vi "BeamformerGUI_GivenFreqs.vi"() -> ()   [LabVIEW 2017]
uses:
  <vilib>/userdefined/High Color/IMAQdx.ctl
  <vilib>/UPVI/lvhdf5/dataset.llb/LVH5D Operation.ctl
  <vilib>/Utility/miscctls.llb/LVRectTypeDef.ctl
  <vilib>/UPVI/lvhdf5/attribute.llb/LVH5A Operation.ctl
  <vilib>/UPVI/lvhdf5/group.llb/H5G_obj_t.ctl
  <vilib>/UPVI/lvhdf5/file.llb/LVH5F Operation.ctl
  15de898c-7c44-4598-bed2-ace033be772a.vi
  <vilib>/UPVI/lvhdf5/identifier.llb/Not an HDF5 Refnum Constant.vi
  <vilib>/UPVI/lvhdf5/common.llb/To HDF5 Ref.vi
  <vilib>/measure/maspectr.llb/FFT Power Spectrum and PSD for 1 Chan.vi
  <vilib>/UPVI/lvhdf5/file.llb/OpenCreateReplace HDF5 File.vi
  <vilib>/UPVI/lvhdf5/utility.llb/Select HDF5 Dialog.vi
  <vilib>/UPVI/lvhdf5/utility.llb/Select HDF5 Dialog (File and Object).vi
  <vilib>/UPVI/lvhdf5/dataset.llb/Simple H5Dwrite (Variant).vi
  <vilib>/UPVI/lvhdf5/attribute.llb/Write Multiple Attributes.vi
  <vilib>/UPVI/lvhdf5/dataset.llb/H5Dclose.vi
  <vilib>/UPVI/lvhdf5/dataset.llb/Write Dataset with Attributes.xnode
  <vilib>/UPVI/lvhdf5/library.llb/HDF5 Ref.ctl
  <vilib>/vision/driver/NI_Vision_Acquisition_Software.lvlib
  <vilib>/Utility/error.llb/Error Cluster From Error Code.vi
  <vilib>/UPVI/lvhdf5/dataset.llb/OpenCreateReplace Dataset by Element Type.vi
  <vilib>/UPVI/lvhdf5/dataspace.llb/H5Sselect_hyperslab.vi
  <vilib>/UPVI/lvhdf5/dataset.llb/H5Dwrite (Variant).vi
  <vilib>/UPVI/lvhdf5/dataset.llb/H5Dget_space.vi
  <vilib>/UPVI/lvhdf5/attribute.llb/private/LVH5AwriteWDTAttrs.vi
  <vilib>/UPVI/lvhdf5/dataspace.llb/H5Sclose.vi
  <vilib>/Utility/VariantDataType/GetClusterInfo.vi
  <vilib>/Utility/VariantDataType/VariantType.lvlib
  <vilib>/Utility/VariantDataType/GetTypeInfo.vi
  <vilib>/UPVI/lvhdf5/attribute.llb/Cluster to Attribute Array.xnode
  <vilib>/measure/NI_MAPro.lvlib
  <vilib>/UPVI/lvhdf5/utility.llb/Select HDF5 Dialog (Object Only).vi
panel:
  in  "Experiment Name 2":string="test_calib"
  out "total_samples":dbl
  out "Data out":dbl[][](array[numeric])
  out "Array":dbl[][](array[numeric])
  in  "stop":bool
  in  "Tab Control":enum32{"Measurement", "Processing"}(tab)
  in  "Distance to array (m)":dbl=0.5
  in  "Take":bool
  in  "Data Directory":path=path "C:/Users/Lino P/Documents/000 - USFQ/TesisProd/data"
  in  "Record Data":bool
  in  "Sampling Freq. (Hz)":dbl=51200.0
  in  "Sampling Time (s)":dbl=10.0
  in  "Experiment Name":string="test_"
  in  "Audio Preview":bool
  out "Image Out":T1(plugin-control)
  in  "Session In":T2 caption="Camera"
  out "Img Ready":bool caption="Capturing Image"
  out "data":dynamicdata(graph)
  in  "Map Threshold":dbl=5.0
  out "Success":bool
  out "Server Running":bool
  out "Processing":bool
  in  "Preview Read Signal":bool
  in  "Scripts Directory":path=path "C:/Users/Lino P/Documents/000 - USFQ/TesisDev/py"
  in  "Lower":dbl=3000.0
  in  "Microphone Geometry":path=path "C:/Users/Lino P/Documents/000 - USFQ/TesisProd/data/xml/16_mics_geom.xml"
  out "Info":string
  out "Warnings":string
  out "Return Code":dbl
  out "Error":bool
  in  "Audio Data File (HDF5)":path=path "C:/Users/Lino P/Documents/000 - USFQ/TesisProd/data/test_exe.h5"
  in  "RunAnalysis":bool
  out "Selected Mic":dbl[](graph)
  out "Frequency Domain":cluster{"f0":dbl, "df":dbl, "magnitude":dbl[]}(graph)
  out "Sampling Freq. (Hz)":dbl
  in  "Higher":dbl=5000.0 caption="high_freq"
  in  "Channel":u16(ring) items=["1", "2", "3", "4", "5", "6", "7", "8", "9", "10", "11", "12", "13", "14", "15", "16"]
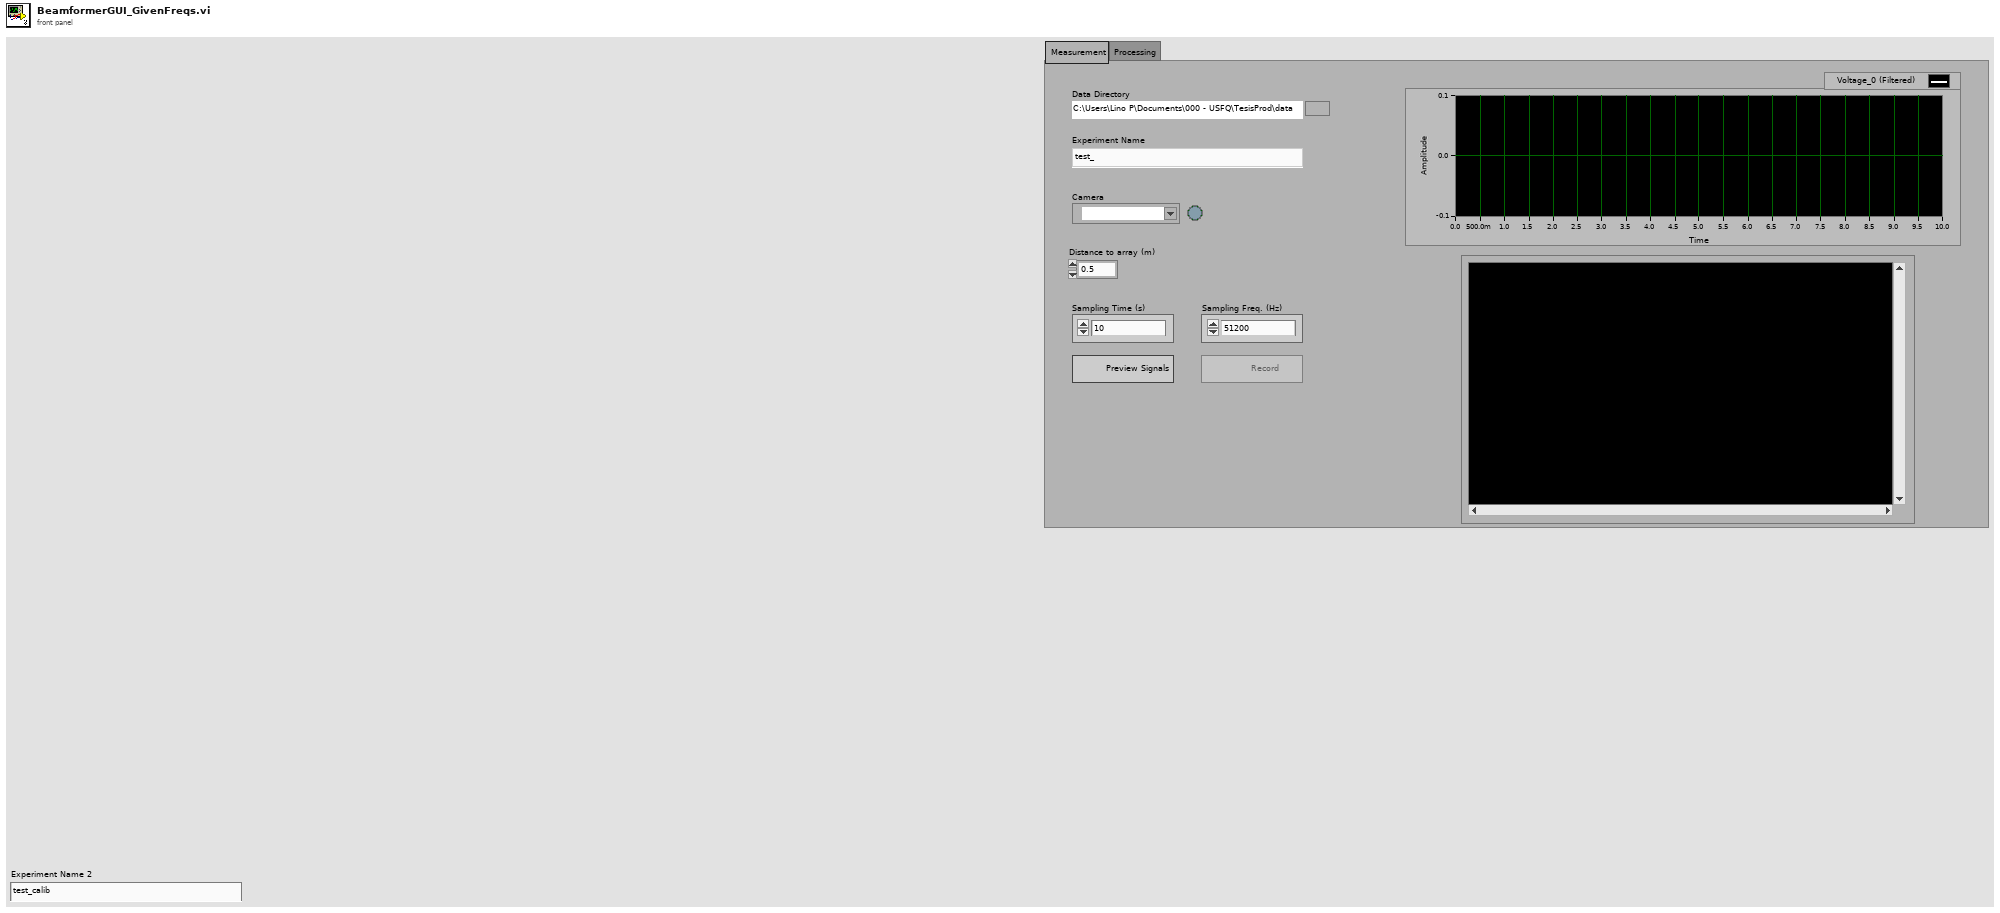
[diagram p1: front panel]
types:
  T1 = typedef "IMAQ Image.ctl" = refnum<image>
  T2 = typedef "IMAQdx.ctl" = refnum<k21>
  T3 = enum8{"Enabled", "Disabled", "Disabled and Grayed Out"}
  T4 = typedef "Image Type" = u32
  T5 = typedef "LVH5D Operation.ctl" = enum16{"open", "replace", "create", "open or create", "create or replace", "create or replace with confirmation"}
  T6 = typedef "LVH5A Operation.ctl" = enum16{"open", "replace", "create", "open or create", "create or replace", "create or replace with confirmation"}
  T7 = typedef "LVRectTypeDef.ctl" = cluster{"Left":i16, "Top":i16, "Right":i16, "Bottom":i16}
  T8 = cluster{"Behavior":enum32{"Invalid", "Default", "Floating", "Floating/Auto-Hide", "Modal"}, "Position":T7, "Center":bool, "Title":string}
  T9 = typedef "LVH5F Operation.ctl" = enum16{"open", "open or create", "create or replace", "create or replace (with confirmation)", "create", "open (read only)"}
  T10 = typedef "H5G_obj_t.ctl" = i32
  T11 = cluster{"Object Types (any)":T10[], "Object Pattern":string}
  T12 = enum32{"Invalid", "Standard", "Closed", "Hidden", "Minimized", "Maximized"}
  T13 = typedef "HDF5 Ref.ctl" = refnum<k1>
  T14 = cluster{"Left":i32, "Top":i32, "Right":i32, "Bottom":i32}
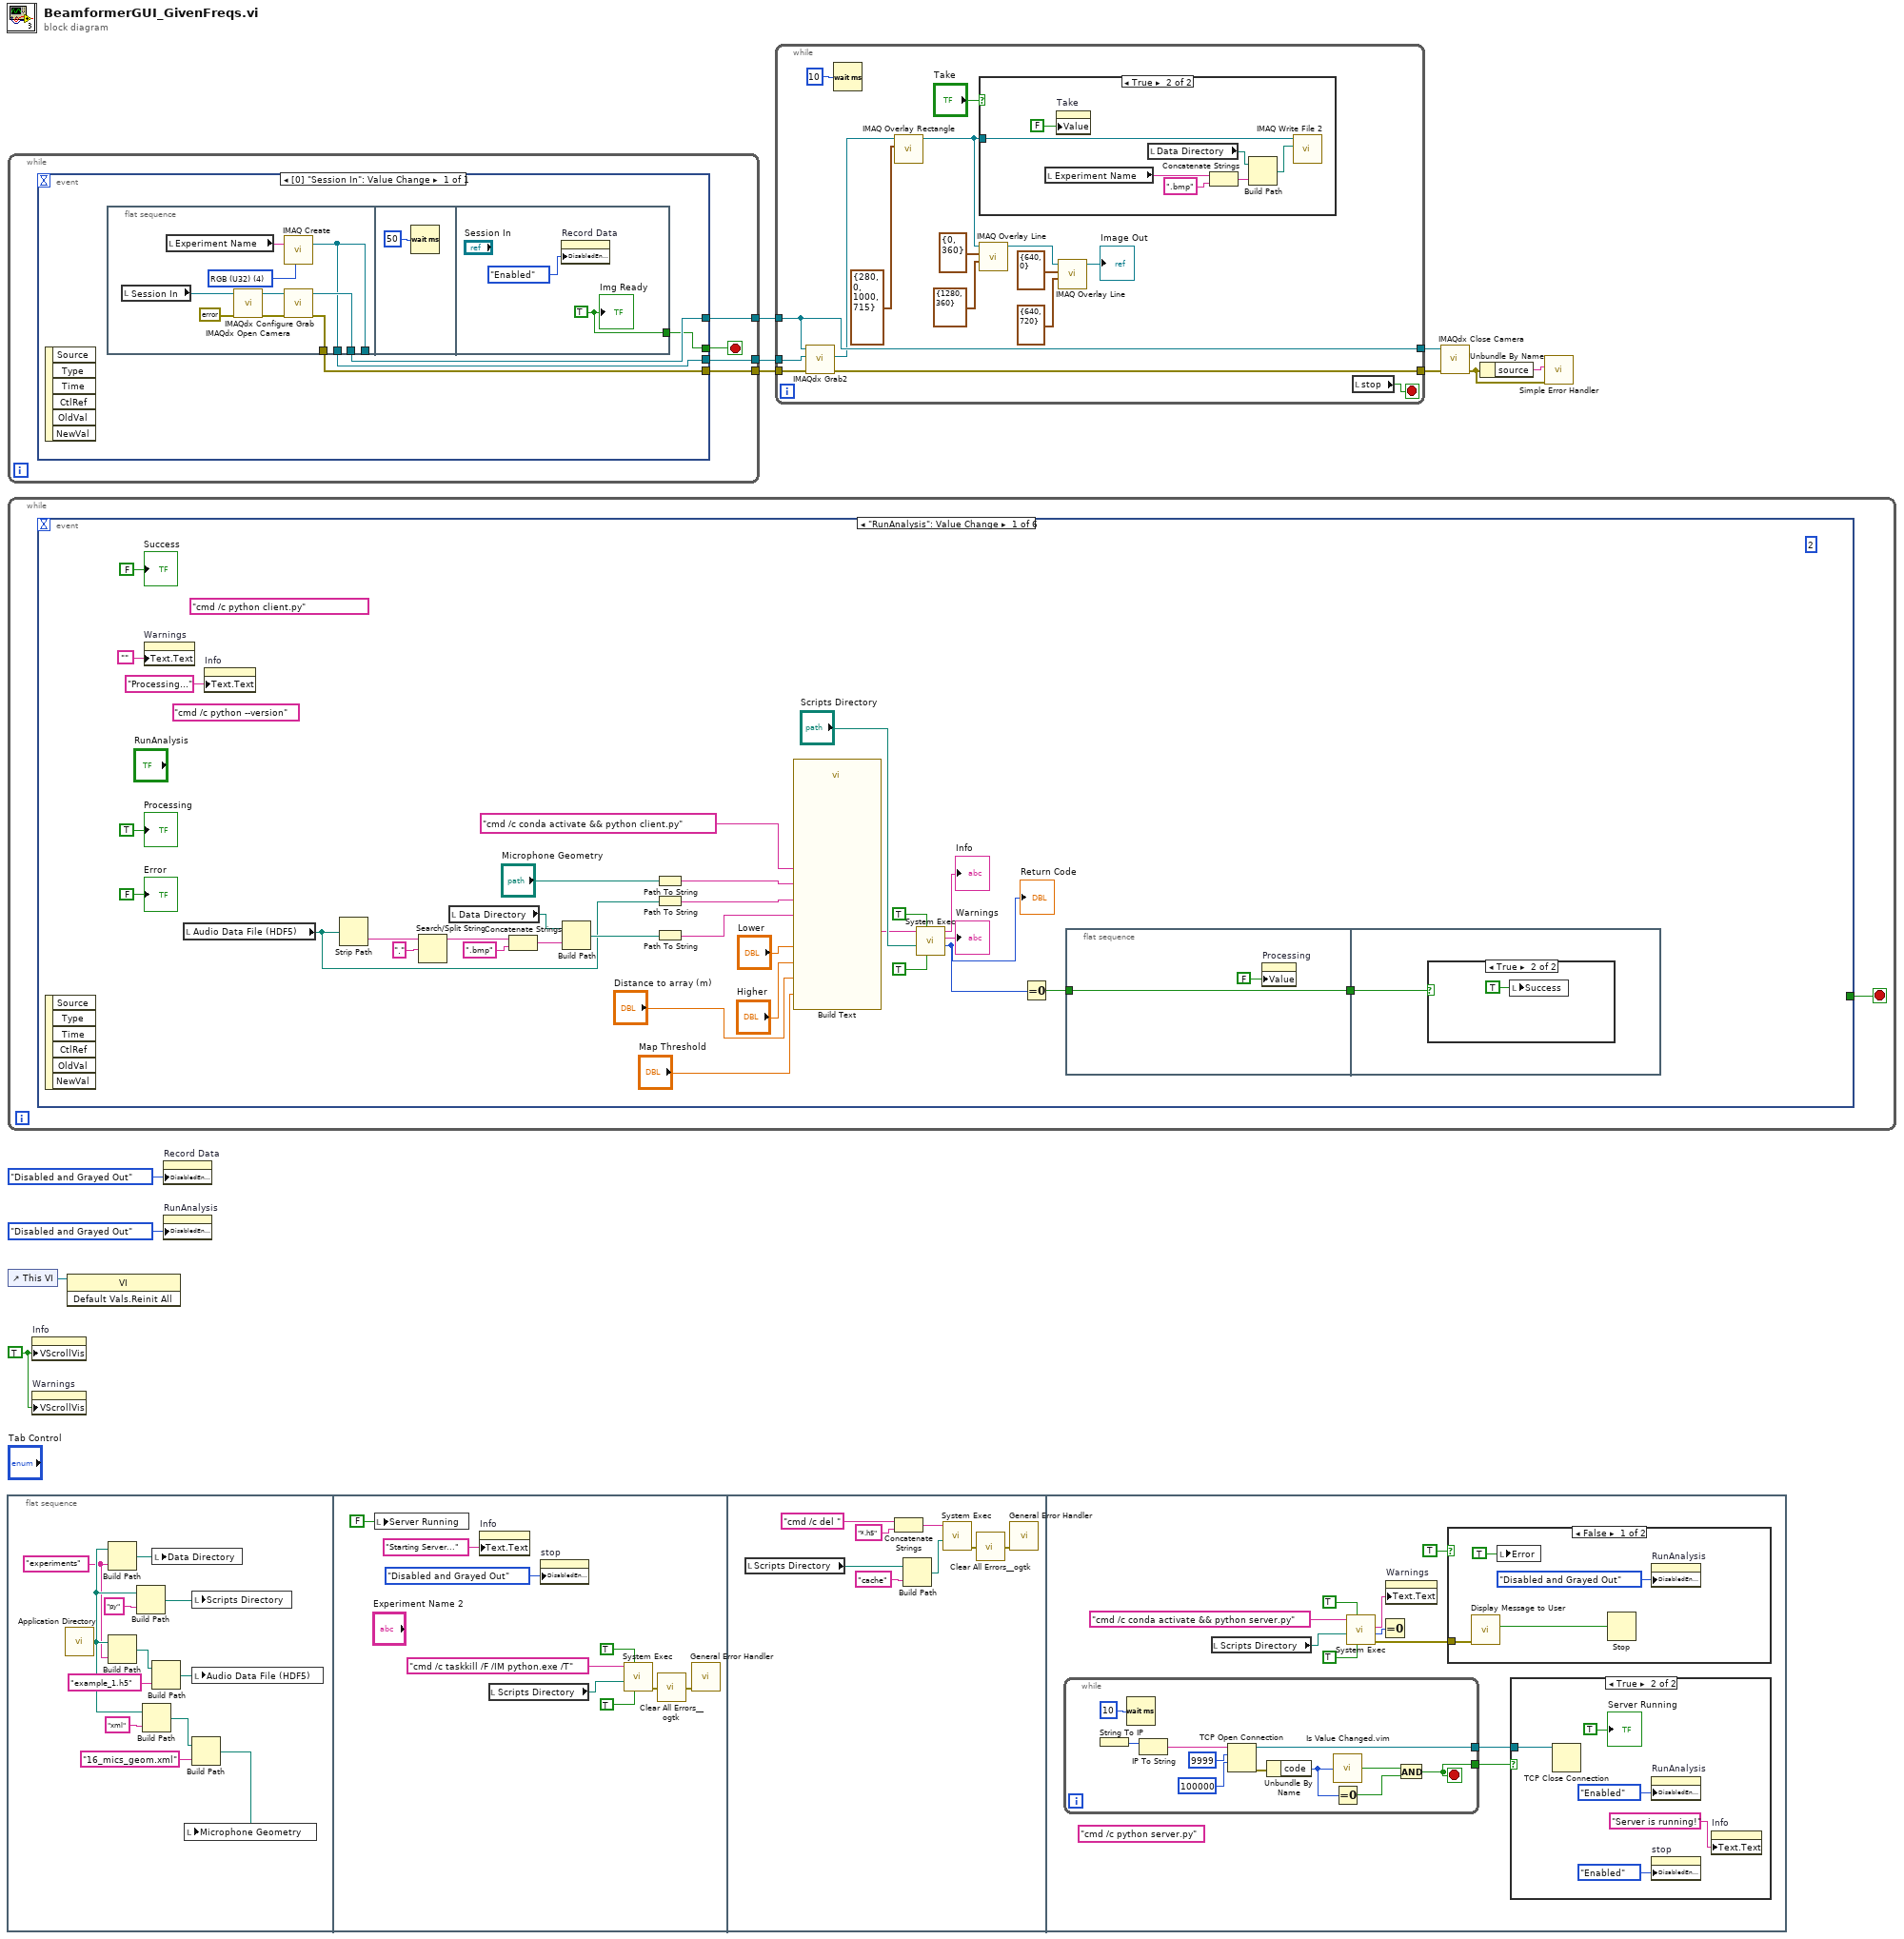
[diagram p0: block diagram]
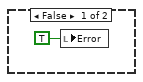
[diagram p5: hidden frame]
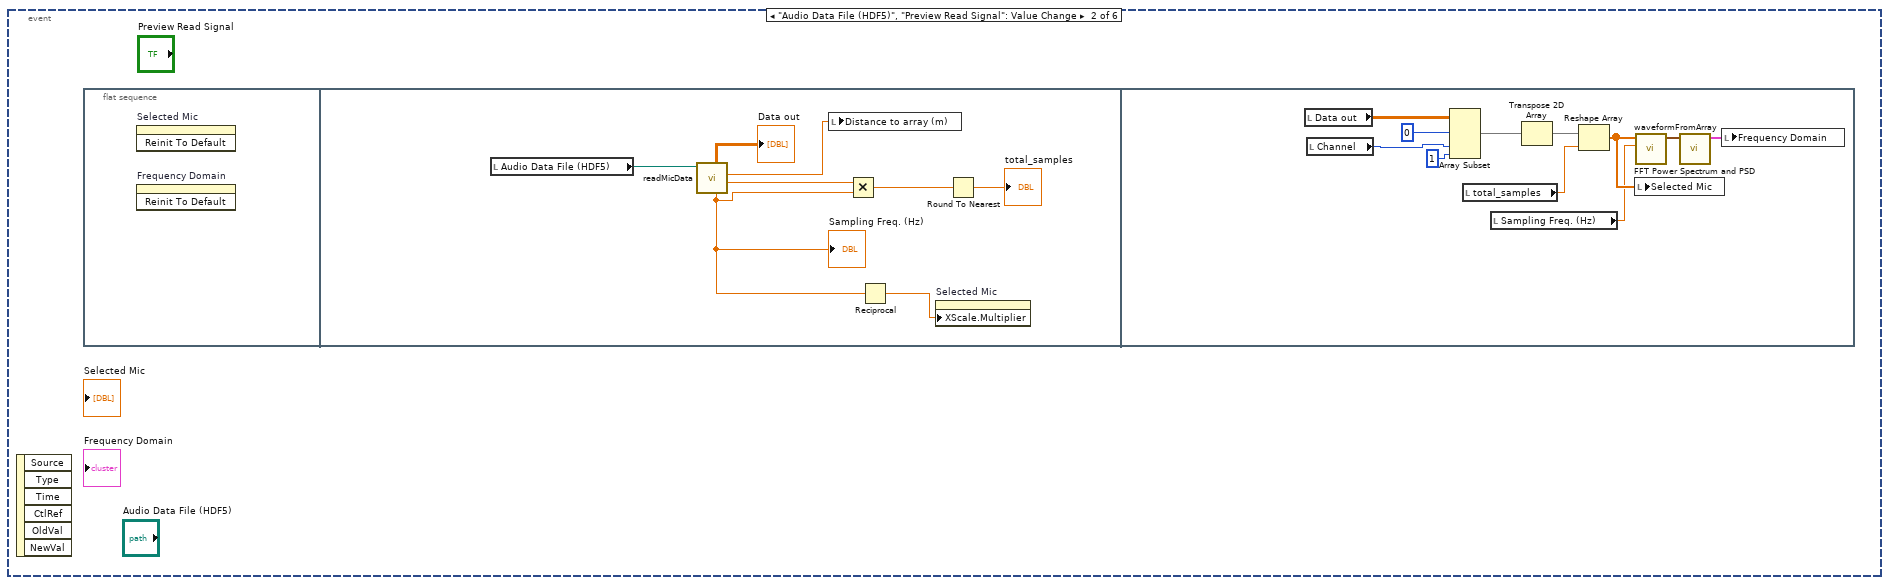
[diagram p6: hidden frame]
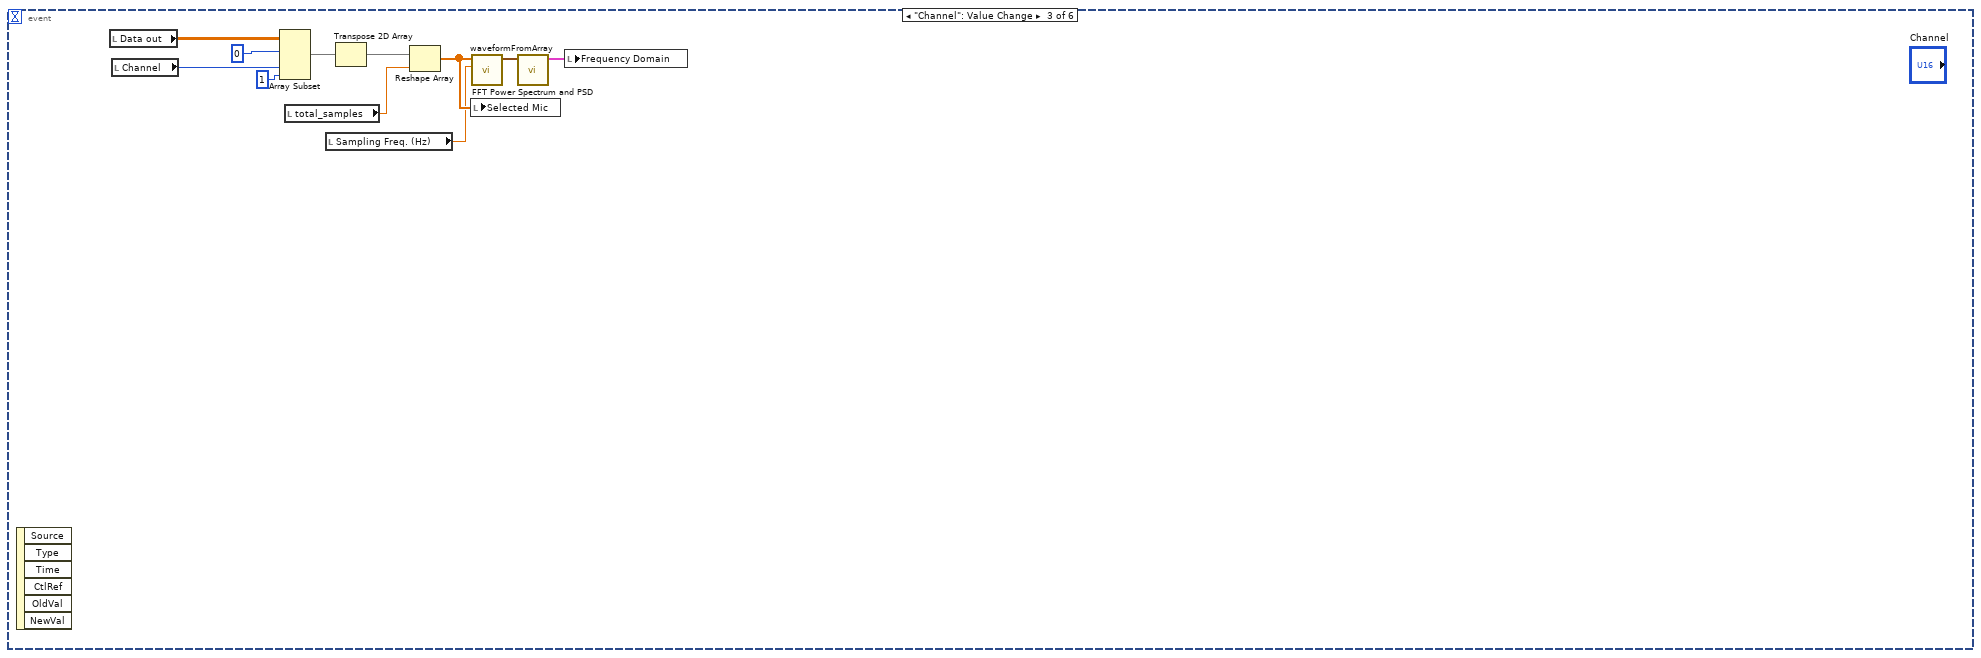
[diagram p7: hidden frame]
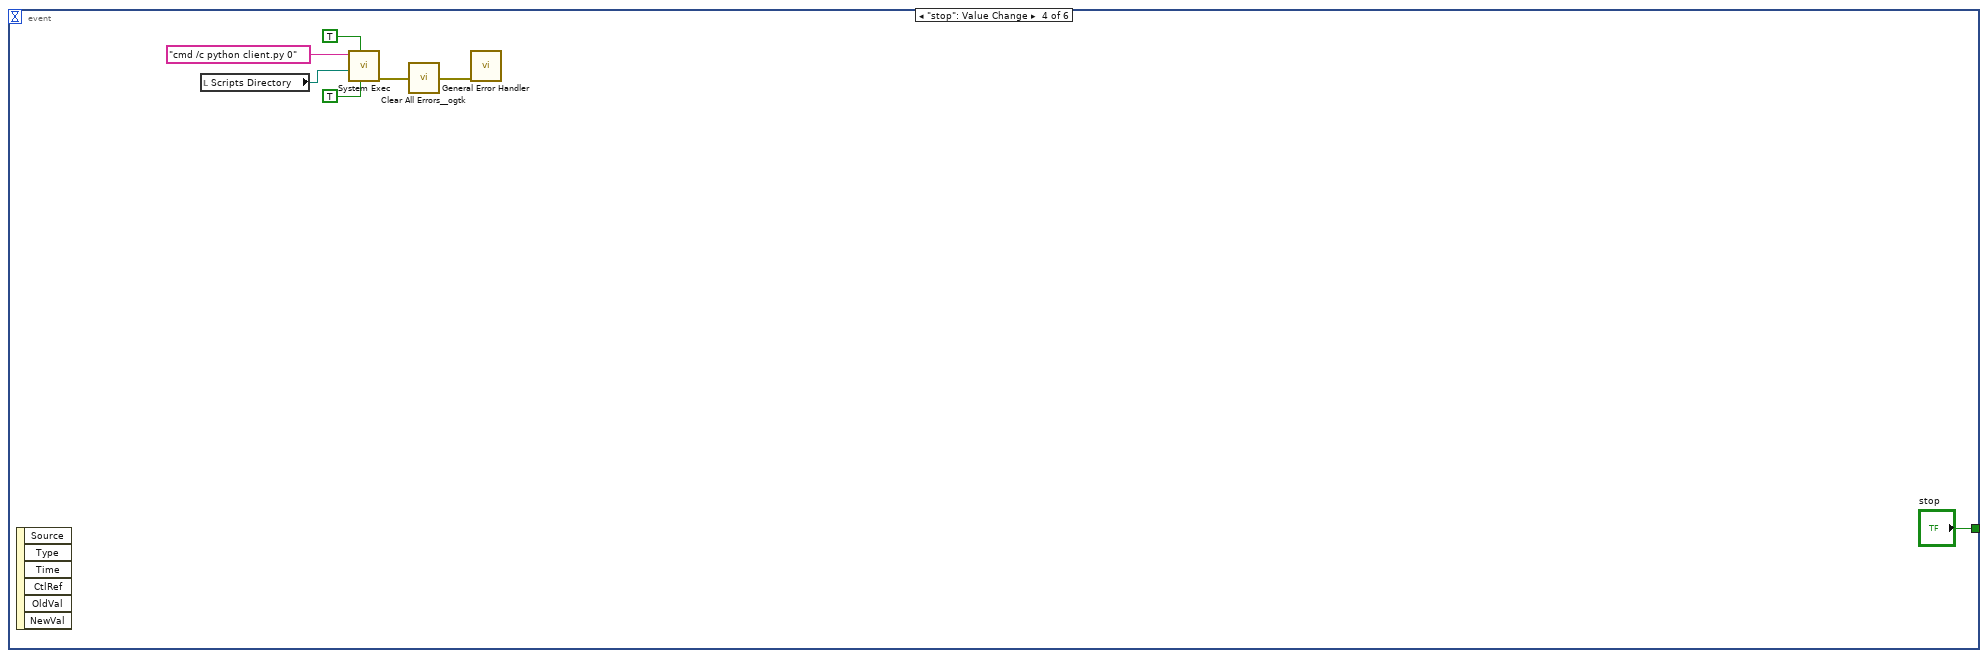
[diagram p8: hidden frame]
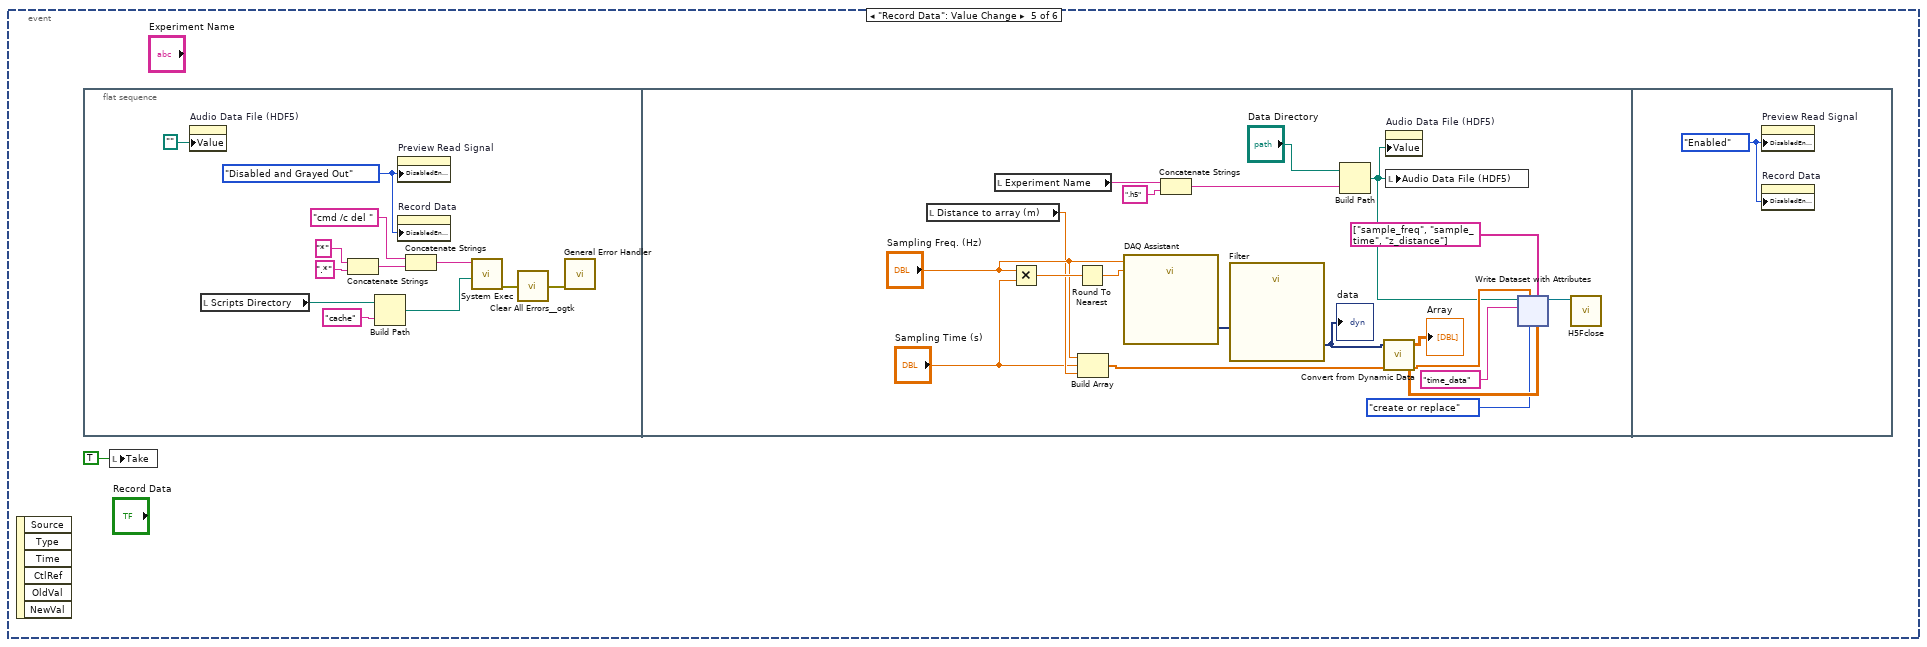
[diagram p9: hidden frame]
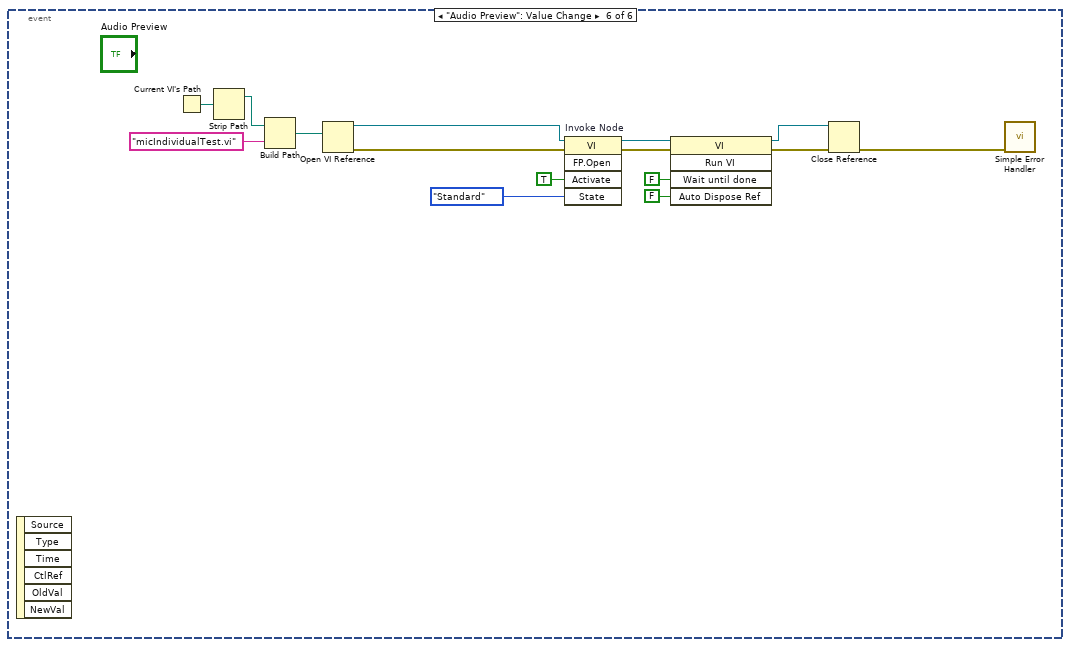
[diagram p10: hidden frame]
diagram:
  w10 = TRUE
  n1 = flat-sequence {
    frame #0 {
      w16 = "experiments" ("name or relative path")
      n2 = call <vilib>:"Application Directory.vi"() -> ("Application Directory"=w19:path)
      n3 = Build Path(base path=w19, name or relative path=w16) -> (appended path=w20:path)
      n4 = Build Path(base path=w19, name or relative path=w16) -> (appended path=w15:path)
      n5 = Build Path(base path=w19, name or relative path="py") -> (appended path=w22:path)
      n6 = Build Path(base path=w19, name or relative path="xml") -> (appended path=w18:path)
      n7 = local write "Data Directory"(w20) -> ()
      n8 = Build Path(base path=w15, name or relative path="example_1.h5") -> (appended path=w13:path)
      n9 = local write "Scripts Directory"(w22) -> ()
      n10 = local write "Audio Data File (HDF5)"(w13) -> ()
      n11 = Build Path(base path=w18, name or relative path="16_mics_geom.xml") -> (appended path=w12:path)
      n12 = local write "Microphone Geometry"(w12) -> ()
    }
    frame #1 {
      n13 = local write "Server Running"(FALSE ("Server Running")) -> ()
      n14 = property on="Info" class="Str"("Text.Text"="Starting Server...") -> ()  [unwired: 2 in, 2 out]
      n15 = local read "Scripts Directory"() -> (w32:path)
      n16 = property on="stop" class="Bool (strict)"("DisabledEnum"=T3."Disabled and Grayed Out" ("Disabled")) -> ()  [unwired: 2 in, 2 out]
      n17 = call <vilib>:"System Exec.vi"("run minimized? (F)"=TRUE, "wait until completion? (T)"=TRUE, "working directory"=w32, "command line"="cmd /c taskkill /F /IM python.exe /T") -> ("error out"=w28:errorcluster)  [unwired: 4 in, 3 out]
      n18 = call <userlib>:"Clear All Errors__ogtk.vi"("Error In"=w28) -> ("Error Out"=w29:errorcluster)  [unwired: 3 in]
      n19 = call <vilib>:"General Error Handler.vi"("error in (no error)"=w29) -> ()  [unwired: 10 in, 5 out]
    }
    frame #2 {
      n20 = local read "Scripts Directory"() -> (w39:path)
      n21 = Concatenate Strings("cmd /c del " ("command line"), "*.h5" ("string")) -> (w36:string)
      n22 = Build Path(base path=w39, name or relative path="cache") -> (appended path=w40:path)
      n23 = call <vilib>:"System Exec.vi"("working directory"=w40, "command line"=w36) -> ("error out"=w38:errorcluster)  [unwired: 6 in, 3 out]
      n24 = call <userlib>:"Clear All Errors__ogtk.vi"("Error In"=w38) -> ("Error Out"=w37:errorcluster)  [unwired: 3 in]
      n25 = call <vilib>:"General Error Handler.vi"("error in (no error)"=w37) -> ()  [unwired: 10 in, 5 out]
    }
    frame #3 {
      (unwired) "cmd /c python server.py" ("command line")
      n26 = while {
        tunnel: [w60] -> w42
        tunnel: [w58] -> w41
        stop <- w60 stop-if-true
        n27 = String To IP() -> (0:w56:u32)  [unwired: 1 in]
        n28 = Wait (ms)(milliseconds to wait=u32 10) -> ()  [unwired: 1 out]
        n29 = IP To String(2:w56) -> (0:w57:string)  [unwired: 1 in]
        n30 = TCP Open Connection(address=w57, remote port or service name=u16 9999, timeout ms (60000)=100000) -> (connection ID=w58:refnum<k5>, error out=w59:errorcluster)  [unwired: 2 in]
        n31 = Unbundle By Name(w59) -> ("code"=w63:i32)
        n32 = call "Is Value Changed.vim"("value"=w63) -> ("changed or first call?"=w61:bool)
        n33 = Equal To 0?(x=w63) -> (x = 0?=w62:bool)
        n34 = And(x=w61, y=w62) -> (x .and. y?=w60:bool)
      }
      n35 = local read "Scripts Directory"() -> (w47:path)
      n36 = call <vilib>:"System Exec.vi"("run minimized? (F)"=TRUE, "wait until completion? (T)"=TRUE, "working directory"=w47, "command line"="cmd /c conda activate && python server.py") -> ("error out"=w49:errorcluster, "return code"=w48:i32, "standard error"=w50:string)  [unwired: 4 in, 1 out]
      n37 = Equal To 0?(x=w48) -> ()  [unwired: 1 out]
      n38 = property on="Warnings" class="Str"("Text.Text"=w50) -> ()  [unwired: 2 in, 2 out]
      n39 = case shown="False" TRUE {
        tunnel: w49 -> [w67 _]
        frame False {
          n40 = call "Display Message to User"("error in (no error)"=w67) -> ("OK"=w68:bool)  [unwired: 9 in, 1 out]
          n41 = local write "Error"(TRUE ("Error")) -> ()
          n42 = Stop(stop? (T)=w68) -> ()
          n43 = property on="RunAnalysis" class="Bool"("DisabledEnum"=T3."Disabled and Grayed Out" ("Disabled")) -> ()  [unwired: 2 in, 2 out]
        }
        frame True {
        }
      }
      n44 = case shown="True" w42 {
        tunnel: w41 -> [_ w54]
        frame False {
        }
        frame True {
          n45 = TCP Close Connection(connection ID=w54) -> ()  [unwired: 2 in, 2 out]
          n46 = property on="RunAnalysis" class="Bool"("DisabledEnum"=T3."Enabled" ("Disabled")) -> ()  [unwired: 2 in, 2 out]
          n47 = property on="stop" class="Bool (strict)"("DisabledEnum"=T3."Enabled" ("Disabled")) -> ()  [unwired: 2 in, 2 out]
          n48 = property on="Info" class="Str"("Text.Text"="Server is running!") -> ()  [unwired: 2 in, 2 out]
          "Server Running" <- TRUE ("Server Running")
        }
      }
    }
  }
  n49 = while {
    tunnel: [w73] -> w5
    tunnel: [w74] -> w4
    tunnel: [w72] -> w1
    stop <- w71 stop-if-true
    n50 = event shown="[0] \"Session In\": Value Change" {
      selector: _ -> [_]
      dyn-events: _ -> [_]
      timeout: _ -> [_]
      tunnel: [w78] -> w74
      tunnel: [w77] -> w73
      tunnel: [w76] -> w72
      tunnel: [w75] -> w71
      event Value Change {
        n51 = event-data() -> ()  [unwired: 1 in, 6 out]
        n52 = flat-sequence {
          tunnel: [w82] -> w78
          tunnel: [w81] -> w77
          tunnel: [w79] -> w76
          tunnel: [w79] -> _
          tunnel: [w90] -> w75
          frame #0 {
            w83 = T4 4 items=["Grayscale (U8)", "Grayscale (I16)", "Grayscale (SGL)", "Complex (CSG)", "RGB (U32)", "HSL (U32)", "RGB (U64)", "Grayscale (U16)"] ("Image Type")
            n53 = local read "Session In"() -> (w87:T2)
            n54 = local read "Experiment Name"() -> (w80:string)
            n55 = call <vilib>:"IMAQdx Open Camera.vi"("error in"=errorcluster {"status"=FALSE, "code"=0, "source"=""}, "Session In"=w87) -> ("error out"=w85:errorcluster, "Session Out"=w86:T2)  [unwired: 8 in]
            n56 = call "IMAQ Create"("Image Name"=w80, "Image Type"=w83) -> ("New Image"=w79:T1)  [unwired: 3 in, 1 out]
            n57 = call <vilib>:"IMAQdx Configure Grab.vi"("error in"=w85, "Session In"=w86) -> ("error out"=w82:errorcluster, "Session Out"=w81:T2)  [unwired: 8 in]
          }
          frame #1 {
            n58 = Wait (ms)(milliseconds to wait=u32 50) -> ()  [unwired: 1 out]
          }
          frame #2 {
            w90 = TRUE
            n59 = property on="Record Data" class="Bool"("DisabledEnum"=T3."Enabled" ("Disabled")) -> ()  [unwired: 2 in, 2 out]
            "Img Ready" <- w90
          }
        }
      }
    }
  }
  n60 = while {
    stop <- w91 stop-if-true
    n61 = event shown="[0] \"RunAnalysis\": Value Change" {
      selector: _ -> [_ _ _ _ _ _]
      dyn-events: _ -> [_ _ _ _ _ _]
      timeout: _ -> [_ _ _ _ _ _]
      tunnel: [_ _ _ "stop" _ _] -> w91
      event "RunAnalysis": Value Change {
        (unwired) "cmd /c python client.py"
        (unwired) 2
        (unwired) "cmd /c python --version" ("command line")
        n62 = event-data() -> ()  [unwired: 1 in, 6 out]
        n63 = property on="Warnings" class="Str"("Text.Text"="") -> ()  [unwired: 2 in, 2 out]
        n64 = local read "Audio Data File (HDF5)"() -> (w95:path)
        n65 = property on="Info" class="Str"("Text.Text"="Processing...") -> ()  [unwired: 2 in, 2 out]
        n66 = Strip Path(path=w95) -> (name=w93:string)  [unwired: 1 out]
        n67 = Search/Split String(string=w93, search string/char (-)=".") -> (substring before match=w92:string)  [unwired: 1 in, 2 out]
        n68 = local read "Data Directory"() -> (w101:path)
        n69 = Concatenate Strings(w92, ".bmp" ("string")) -> (w100:string)
        n70 = Build Path(base path=w101, name or relative path=w100) -> (appended path=w98:path)
        n71 = Path To String(path="Microphone Geometry") -> (string=w117:string)
        n72 = Path To String(path=w95) -> (string=w116:string)
        n73 = Path To String(path=w98) -> (string=w110:string)
        n74 = call "Build Text"("image"=w110, "high_freq"="Higher", "thresh"="Map Threshold", "cmd"="cmd /c conda activate && python client.py", "mic_geo"=w117, "data"=w116, "low_freq"="Lower", "z_distance"="Distance to array (m)") -> ("Result"=w112:string)  [unwired: 6 in, 1 out]
        n75 = call <vilib>:"System Exec.vi"("run minimized? (F)"=TRUE, "wait until completion? (T)"=TRUE, "working directory"="Scripts Directory", "command line"=w112) -> ("return code"=w114:i32, "standard error"=→"Warnings":string, "standard output"=→"Info":string)  [unwired: 4 in, 1 out]
        "Return Code" <- w114
        n76 = Equal To 0?(x=w114) -> (x = 0?=w108:bool)
        n77 = flat-sequence {
          tunnel: w108 -> [w124]
          tunnel: [w124] -> w107
          tunnel: w107 -> [w125]
          frame #0 {
            n78 = property on="Processing" class="Bool (strict)"("Value"=FALSE ("Processing")) -> ()  [unwired: 2 in, 2 out]
          }
          frame #1 {
            n79 = case shown="True" w125 {
              frame False {
                n80 = local write "Error"(TRUE ("Error")) -> ()
              }
              frame True {
                n81 = local write "Success"(TRUE ("Success")) -> ()
              }
            }
          }
        }
        "Processing" <- TRUE
        "Error" <- FALSE ("Error")
        "Success" <- FALSE ("Success\nSuccess")
      }
      event "Audio Data File (HDF5)", "Preview Read Signal": Value Change {
        n82 = event-data() -> ()  [unwired: 1 in, 6 out]
        n83 = flat-sequence {
          frame #0 {
            n84 = invoke on="Selected Mic" class="WFGraph (strict)" method="Reinit To Default"() -> ()  [unwired: 3 in, 3 out]
            n85 = invoke on="Frequency Domain" class="WFGraph (strict)" method="Reinit To Default"() -> ()  [unwired: 3 in, 3 out]
          }
          frame #1 {
            n86 = local read "Audio Data File (HDF5)"() -> (w128:path)
            n87 = call "readMicData.vi"("HDF5 Path or Ref"=w128) -> ("sample_time"=w132:dbl, "z_distance"=w130:dbl, "sample_freq"=w133:dbl, "Data out"=→"Data out":dbl[][])  [unwired: 5 in, 2 out]
            "Sampling Freq. (Hz)" <- w133
            n88 = local write "Distance to array (m)"(w130) -> ()
            n89 = Multiply(x=w132, y=w133) -> (x*y=w131:dbl)
            n90 = Reciprocal(x=w133) -> (1/x=w129:dbl)
            n91 = property on="Selected Mic" class="WFGraph (strict)"("XScale.Multiplier"=w129) -> ()  [unwired: 2 in, 2 out]
            n92 = Round To Nearest(number=w131) -> (nearest integer value=→"total_samples":dbl)
          }
          frame #2 {
            n93 = local read "Data out"() -> (w143:dbl[][])
            n94 = local read "Channel"() -> (w142:u16)
            n95 = Array Subset(array=w143, index (row)=0 ("index"), index (col)=w142, length (col)=1 ("length")) -> (w144:dbl[][])  [unwired: 1 in]
            n96 = local read "total_samples"() -> (w138:dbl)
            n97 = local read "Sampling Freq. (Hz)"() -> (w139:dbl)
            n98 = Transpose 2D Array(2D array=w144) -> (transposed array=w145:dbl[][])
            n99 = Reshape Array(w145, w138) -> (w140:dbl[])
            n100 = local write "Selected Mic"(w140) -> ()
            n101 = call "waveformFromArray.vi"("sample_freq"=w139, "Array"=w140) -> ("waveform"=w146:waveform(dbl))  [unwired: 9 in]
            n102 = call-poly <vilib>:"FFT Power Spectrum and PSD.vi"("time signal"=w146) -> ("Power Spectrum / PSD"=w141:cluster{"f0":dbl, "df":dbl, "magnitude":dbl[]})  [unwired: 7 in, 3 out]
            n103 = local write "Frequency Domain"(w141) -> ()
          }
        }
      }
      event "Channel": Value Change {
        n104 = event-data() -> ()  [unwired: 1 in, 6 out]
        n105 = local read "Data out"() -> (w154:dbl[][])
        n106 = local read "Channel"() -> (w153:u16)
        n107 = Array Subset(array=w154, index (row)=0 ("index"), index (col)=w153, length (col)=1 ("length")) -> (w155:dbl[][])  [unwired: 1 in]
        n108 = local read "total_samples"() -> (w147:dbl)
        n109 = local read "Sampling Freq. (Hz)"() -> (w148:dbl)
        n110 = Transpose 2D Array(2D array=w155) -> (transposed array=w156:dbl[][])
        n111 = Reshape Array(w156, w147) -> (w149:dbl[])
        n112 = local write "Selected Mic"(w149) -> ()
        n113 = call "waveformFromArray.vi"("sample_freq"=w148, "Array"=w149) -> ("waveform"=w157:waveform(dbl))  [unwired: 9 in]
        n114 = call-poly <vilib>:"FFT Power Spectrum and PSD.vi"("time signal"=w157) -> ("Power Spectrum / PSD"=w152:cluster{"f0":dbl, "df":dbl, "magnitude":dbl[]})  [unwired: 7 in, 3 out]
        n115 = local write "Frequency Domain"(w152) -> ()
      }
      event "stop": Value Change {
        n116 = event-data() -> ()  [unwired: 1 in, 6 out]
        n117 = local read "Scripts Directory"() -> (w163:path)
        n118 = call <vilib>:"System Exec.vi"("run minimized? (F)"=TRUE, "wait until completion? (T)"=TRUE, "working directory"=w163, "command line"="cmd /c python client.py 0") -> ("error out"=w158:errorcluster)  [unwired: 4 in, 3 out]
        n119 = call <userlib>:"Clear All Errors__ogtk.vi"("Error In"=w158) -> ("Error Out"=w159:errorcluster)  [unwired: 3 in]
        n120 = call <vilib>:"General Error Handler.vi"("error in (no error)"=w159) -> ()  [unwired: 10 in, 5 out]
      }
      event "Record Data": Value Change {
        n121 = event-data() -> ()  [unwired: 1 in, 6 out]
        n122 = flat-sequence {
          frame #0 {
            w176 = T3."Disabled and Grayed Out" ("Disabled")
            n123 = property on="Audio Data File (HDF5)" class="Path"("Value"=path "") -> ()  [unwired: 2 in, 2 out]
            n124 = local read "Scripts Directory"() -> (w168:path)
            n125 = Concatenate Strings("*" ("string"), ".*" ("string")) -> (w170:string)
            n126 = Build Path(base path=w168, name or relative path="cache") -> (appended path=w167:path)
            n127 = property on="Preview Read Signal" class="Bool"("DisabledEnum"=w176) -> ()  [unwired: 2 in, 2 out]
            n128 = property on="Record Data" class="Bool"("DisabledEnum"=w176) -> ()  [unwired: 2 in, 2 out]
            n129 = Concatenate Strings("cmd /c del " ("command line"), w170) -> (w173:string)
            n130 = call <vilib>:"System Exec.vi"("working directory"=w167, "command line"=w173) -> ("error out"=w171:errorcluster)  [unwired: 6 in, 3 out]
            n131 = call <userlib>:"Clear All Errors__ogtk.vi"("Error In"=w171) -> ("Error Out"=w172:errorcluster)  [unwired: 3 in]
            n132 = call <vilib>:"General Error Handler.vi"("error in (no error)"=w172) -> ()  [unwired: 10 in, 5 out]
          }
          frame #1 {
            n133 = local read "Distance to array (m)"() -> (w192:dbl)
            n134 = local read "Experiment Name"() -> (w182:string)
            n135 = Multiply(x="Sampling Freq. (Hz)", y="Sampling Time (s)") -> (x*y=w194:dbl)
            n136 = Round To Nearest(number=w194) -> (nearest integer value=w195:dbl)
            n137 = Build Array("Sampling Freq. (Hz)", "Sampling Time (s)", w192) -> (w189:dbl[])
            n138 = call "DAQ Assistant"("rate"="Sampling Freq. (Hz)", "number of samples"=w195) -> ("data"=w179:dynamicdata)  [unwired: 15 in, 2 out]
            n139 = Concatenate Strings(w182, ".h5" ("string")) -> (w181:string)
            n140 = call "Filter"("Signal"=w179) -> ("Filtered Signal"=w178:dynamicdata)  [unwired: 9 in, 1 out]
            "data" <- w178
            n141 = Build Path(base path="Data Directory", name or relative path=w181) -> (appended path=w180:path)
            n142 = call "Convert from Dynamic Data"("Dynamic Data Type"=w178) -> ("Array"=w190:dbl[][])  [unwired: 3 in]
            "Array" <- w190
            n143 = property on="Audio Data File (HDF5)" class="Path"("Value"=w180) -> ()  [unwired: 2 in, 2 out]
            n144 = local write "Audio Data File (HDF5)"(w180) -> ()
            n145 = xnode "Write Dataset with Attributes"("Dataset Path"="time_data", "operation (open or create)"=LVH5D_Operation."create or replace", "HDF5 Path or Ref"=w180, "Attribute Name(s)"=string[] ["sample_freq", "sample_time", "z_distance"], "Attribute Value(s)"=w189, "Data"=w190) -> ("HDF5 Ref out"=w187:T13)  [unwired: 2 in, 2 out]
            n146 = call <vilib>:"H5Fclose.vi"("HDF5 Ref"=w187) -> ()  [unwired: 8 in, 1 out]
          }
          frame #2 {
            w490 = T3."Enabled" ("Disabled")
            n147 = property on="Preview Read Signal" class="Bool"("DisabledEnum"=w490) -> ()  [unwired: 2 in, 2 out]
            n148 = property on="Record Data" class="Bool"("DisabledEnum"=w490) -> ()  [unwired: 2 in, 2 out]
          }
        }
        n149 = local write "Take"(TRUE ("Take")) -> ()
      }
      event "Audio Preview": Value Change {
        n150 = event-data() -> ()  [unwired: 1 in, 6 out]
        n151 = Current VI's Path() -> (path=w496:path)
        n152 = Strip Path(path=w496) -> (stripped path=w495:path)  [unwired: 1 out]
        n153 = Build Path(base path=w495, name or relative path="micIndividualTest.vi") -> (appended path=w493:path)
        n154 = Open VI Reference(vi path=w493) -> (vi reference=w492:refnum<vi>, error out=w491:errorcluster)  [unwired: 1 in, 4 out]
        n155 = invoke on="Invoke Node" class="VI" method="FP.Open"(reference=w492, error in=w491, "Activate"=TRUE ("Activate?"), "State"=T12."Standard") -> (reference out=w499:refnum<vi>, error out=w500:errorcluster)  [unwired: 1 in, 3 out]
        n156 = invoke class="VI" method="Run VI"(reference=w499, error in=w500, "Wait until done"=FALSE ("Wait Until Done"), "Auto Dispose Ref"=FALSE ("Auto Dispose Reference")) -> (reference out=w498:refnum<vi>, error out=w497:errorcluster)  [unwired: 1 in, 3 out]
        n157 = Close Reference(reference=w498, error in (no error)=w497) -> (error out=w505:errorcluster)
        n158 = call <vilib>:"Simple Error Handler.vi"("error in (no error)"=w505) -> ()  [unwired: 1 in, 8 out]
      }
    }
  }
  n159 = control-ref of="This VI"() -> (w11:refnum<vi>)
  n160 = property on="Info" class="Str"("VScrollVis"=w10) -> ()  [unwired: 2 in, 2 out]
  n161 = property on="Warnings" class="Str"("VScrollVis"=w10) -> ()  [unwired: 2 in, 2 out]
  n162 = invoke class="VI" method="Default Vals.Reinit All"(reference=w11) -> ()  [unwired: 2 in, 3 out]
  n163 = property on="Record Data" class="Bool"("DisabledEnum"=T3."Disabled and Grayed Out" ("Disabled")) -> ()  [unwired: 2 in, 2 out]
  n164 = property on="RunAnalysis" class="Bool"("DisabledEnum"=T3."Disabled and Grayed Out" ("Disabled")) -> ()  [unwired: 2 in, 2 out]
  n165 = while {
    tunnel: w4 -> [w521]
    tunnel: [w520] -> w6
    tunnel: w5 -> [w518]
    tunnel: w1 -> [w519]
    tunnel: [w518] -> w9
    stop <- w516 stop-if-true
    n166 = call <vilib>:"IMAQdx Grab2.vi"("error in"=w521, "Image In"=w519, "Session In"=w518) -> ("error out"=w520:errorcluster, "Image Out"=w513:T1)  [unwired: 5 in, 2 out]
    n167 = Wait (ms)(milliseconds to wait=u32 10) -> ()  [unwired: 1 out]
    n168 = call "IMAQ Overlay Rectangle"("Rectangle"=T14 {"Left"=280, "Top"=0, "Right"=1000, "Bottom"=715}, "Image"=w513) -> ("Image Out"=w512:T1)  [unwired: 8 in, 1 out]
    n169 = case shown="True" "Take" {
      tunnel: w512 -> [_ w522]
      frame False {
      }
      frame True {
        n170 = local read "Experiment Name"() -> (w523:string)
        n171 = property on="Take" class="Bool (strict)"("Value"=FALSE ("Take")) -> ()  [unwired: 2 in, 2 out]
        n172 = local read "Data Directory"() -> (w527:path)
        n173 = Concatenate Strings(w523, ".bmp" ("string")) -> (w524:string)
        n174 = Build Path(base path=w527, name or relative path=w524) -> (appended path=w528:path)
        n175 = call-poly "IMAQ Write File 2"("File Path"=w528, "Image"=w522) -> ()  [unwired: 8 in, 2 out]
      }
    }
    n176 = call "IMAQ Overlay Line"("End Point"=cluster{"X":i32, "Y":i32} {"X"=1280, "Y"=360}, "Start Point"=cluster{"X":i32, "Y":i32} {"X"=0, "Y"=360}, "Image"=w512) -> ("Image Out"=w509:T1)  [unwired: 7 in, 1 out]
    n177 = call "IMAQ Overlay Line"("End Point"=cluster{"X":i32, "Y":i32} {"X"=640, "Y"=720}, "Start Point"=cluster{"X":i32, "Y":i32} {"X"=640, "Y"=0}, "Image"=w509) -> ("Image Out"=→"Image Out":T1)  [unwired: 7 in, 1 out]
    n178 = local read "stop"() -> (w516:bool)
  }
  n179 = call <vilib>:"IMAQdx Close Camera.vi"("error in"=w6, "Session In"=w9) -> ("error out"=w8:errorcluster)  [unwired: 9 in]
  n180 = Unbundle By Name(w8) -> ("source"=w7:string)
  n181 = call <vilib>:"Simple Error Handler.vi"("error source (\" \")"=w7, "error in (no error)"=w8) -> ()  [unwired: 3 in, 5 out]
